vi "MenuHandler.vi"(5 "tree control":refnum<vi>, 7 "main queue":refnum<queue>, 8 "error in":errorcluster, 9 "parameters":variant, 10 "menu string":string, 11 "DMM Instrument":refnum<class "DMM Instrument.lvclass">) -> (0 "error out":errorcluster, 1 "refresh tree?":bool, 2 "Unhandled":bool, 3 "DMM Instrument out":refnum<class "DMM Instrument.lvclass">)   [LabVIEW 2025, in "DMM.lvlib" / "DMM Instrument.lvclass"]
doc: "Copyright 2017 National Instruments Corporation\n\nLicensed under the Apache License, Version 2.0 (the \"License\"); you may not use this file except in compliance with the License. You may obtain a copy of the License at http://www.apache.org/licenses/LICENSE-2.0\nUnless required by applicable law or agreed to in writing, software distributed under the License is distributed on an \"AS IS\" BASIS, WITHOUT WARRANTIES OR CONDITIONS OF ANY KIND, either express or implied. See the License for the specific language governing permissions and limitations under the License."
uses:
  DMM Instrument.lvclass
  DMM Instrument.lvclass/DMM Instrument.ctl
  Users/Public/Documents/Sandia National Labs/TSS Plugin/Abstract Engine.lvlibp/Plugin/Abstract/Abstract Instrument/Abstract Instrument.lvclass
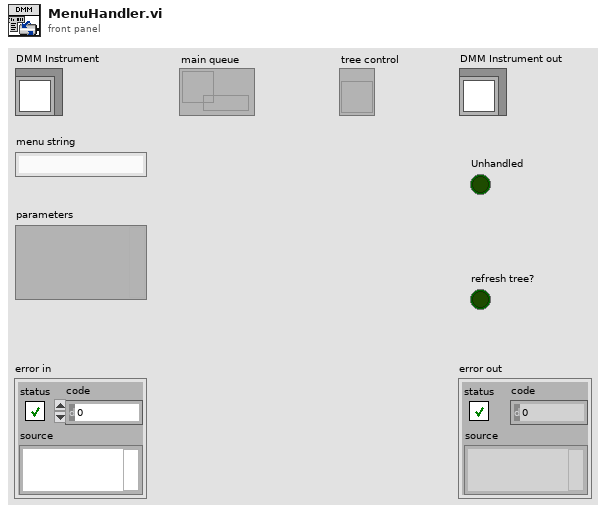
[diagram p1: front panel]
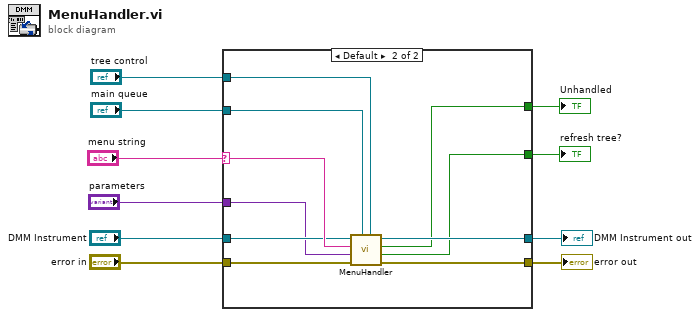
[diagram p0: block diagram]
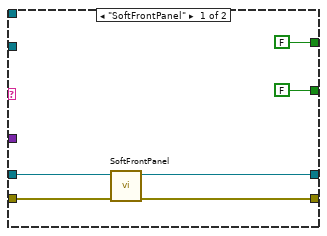
[diagram p2: hidden frame]
diagram:
  n1 = case shown="Default" "menu string" {
    selector: "menu string" -> [_ w24]
    tunnel: [w11 w26] -> w9
    tunnel: [w13 w25] -> w8
    tunnel: [FALSE ("Unhandled") w23] -> w2
    tunnel: [FALSE ("refresh tree?") w22] -> w1
    tunnel: "error in" -> [w12 w20]
    tunnel: "DMM Instrument" -> [w14 w21]
    tunnel: "parameters" -> [_ w19]
    tunnel: "main queue" -> [_ w18]
    tunnel: "tree control" -> [_ w17]
    frame "SoftFrontPanel" {
      n2 = call "SoftFrontPanel.vi"("error in (no error)"=w12, "DMM Instrument"=w14) -> ("error out"=w11:errorcluster, "DMM Instrument out"=w13:refnum<class "DMM Instrument.lvclass">)  [unwired: 8 in]
    }
    frame Default {
      n3 = call-parent "MenuHandler.vi"("tree control"=w17, "main queue"=w18, "error in"=w20, "parameters"=w19, "menu string"=w24, "CEF_serializable node in"=w21) -> ("error out"=w26:errorcluster, "refresh tree?"=w22:bool, "Unhandled"=w23:bool, "CEF_serializable node out"=w25:refnum<class "DMM Instrument.lvclass">)  [unwired: 2 in]
    }
  }
  "error out" <- w9
  "DMM Instrument out" <- w8
  "Unhandled" <- w2
  "refresh tree?" <- w1
